vi "题目五.vi"() -> ()   [LabVIEW 2017]
panel:
  in  "停止":bool
  out "恭喜":bool
  out "通过":bool
  out "警告":bool
  in  "分数":dbl
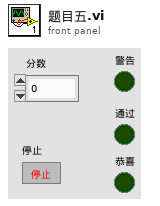
[diagram p1: front panel]
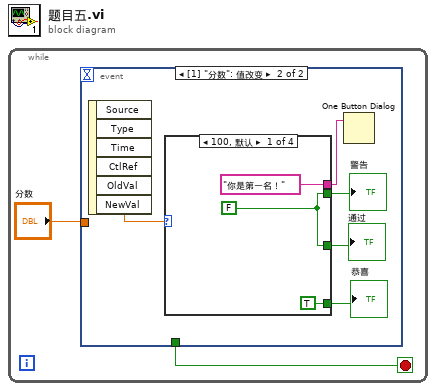
[diagram p0: block diagram]
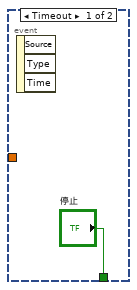
[diagram p2: hidden frame]
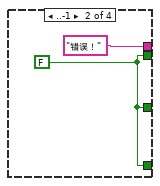
[diagram p3: hidden frame]
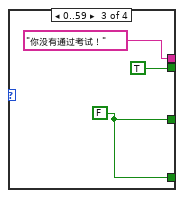
[diagram p4: hidden frame]
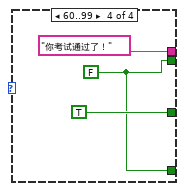
[diagram p5: hidden frame]
diagram:
  n1 = while {
    stop <- w1 stop-if-true
    n2 = event shown="[1] \"分数\": 值改变" {
      selector: _ -> [_ _]
      dyn-events: _ -> [_ _]
      timeout: _ -> [_ _]
      tunnel: "分数" -> [_ _]
      tunnel: ["停止" _] -> w1
      event Timeout {
        n3 = event-data() -> ()  [unwired: 1 in, 3 out]
      }
      event "分数": Value Change {
        n4 = event-data() -> ("NewVal"=w4:dbl)  [unwired: 1 in, 5 out]
        n5 = case shown="100, 默认" w4 {
          tunnel: [w9 w12 TRUE w17] -> w8
          tunnel: [w9 w12 w14 TRUE] -> w7
          tunnel: [TRUE w12 w14 w17] -> w6
          tunnel: ["你是第一名！" "错误！" "你没有通过考试！" "你考试通过了！"] -> w5
          frame 100, Default {
            w9 = FALSE
          }
          frame ..-1 {
            w12 = FALSE
          }
          frame 0..59 {
            w14 = FALSE
          }
          frame 60..99 {
            w17 = FALSE
          }
        }
        "警告" <- w8
        "通过" <- w7
        "恭喜" <- w6
        n6 = One Button Dialog(message=w5) -> ()  [unwired: 1 in, 1 out]
      }
    }
  }
